vi "Close PolarizationProcessorSDK.vi"(8 "error in (no error)":errorcluster, 11 "PolarizationProcessorSDK reference":refnum<k24>) -> (0 "error out":errorcluster)   [LabVIEW 2015]
uses:
  C:/code/Host/Installer/Scientific Camera Interfaces/LabVIEW/32_bit/Library_X86/Thorlabs.TSI.PolarizationProcessor.dll
  code/Host/Installer/Scientific Camera Interfaces/LabVIEW/32_bit/Library_X86/Thorlabs.TSI.PolarizationProcessor.dll
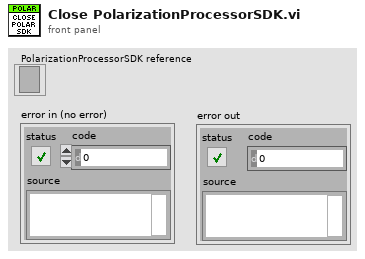
[diagram p1: front panel]
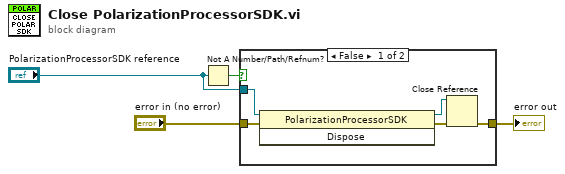
[diagram p0: block diagram]
diagram:
  n1 = Not A Number/Path/Refnum?(number/path/refnum="PolarizationProcessorSDK reference") -> (NaN/Path/Refnum?=w2:bool)
  n2 = case shown="False" w2 {
    tunnel: "error in (no error)" -> [w9 w10]
    tunnel: [w6 w10] -> w3
    tunnel: "PolarizationProcessorSDK reference" -> [w5 _]
    frame False {
      n3 = invoke class="PolarizationProcessorSDK" method="Dispose"(reference=w5, error in=w9) -> (reference out=w7:refnum<k24>, error out=w8:errorcluster)  [unwired: 1 in, 1 out]
      n4 = Close Reference(reference=w7, error in (no error)=w8) -> (error out=w6:errorcluster)
    }
    frame True {
    }
  }
  "error out" <- w3
